vi "IQR Filter 3.vi"(9 "Z Values":dbl[](array[numeric]), 10 "Y Values":dbl[](array[numeric]), 11 "X Values":dbl[](array[numeric])) -> (1 "Z Vector":dbl[](array[numeric]), 2 "Y Vector":dbl[](array[numeric]), 3 "X Value":dbl[](array[numeric]))   [LabVIEW 2017]
uses:
  <vilib>/Analysis/NI_AALBase.lvlib
panel:
  out "Outliers":i32[](array[numeric])
  out "Higher Inner Fence":dbl
  out "Lower Inner Fence":dbl
  out "Interquartile Range":dbl
  out "Q1":dbl format="%.10f"
  out "median":dbl format="%.10f"
  out "Q3":dbl format="%.10f"
  out "X Histogram":T1(graph)
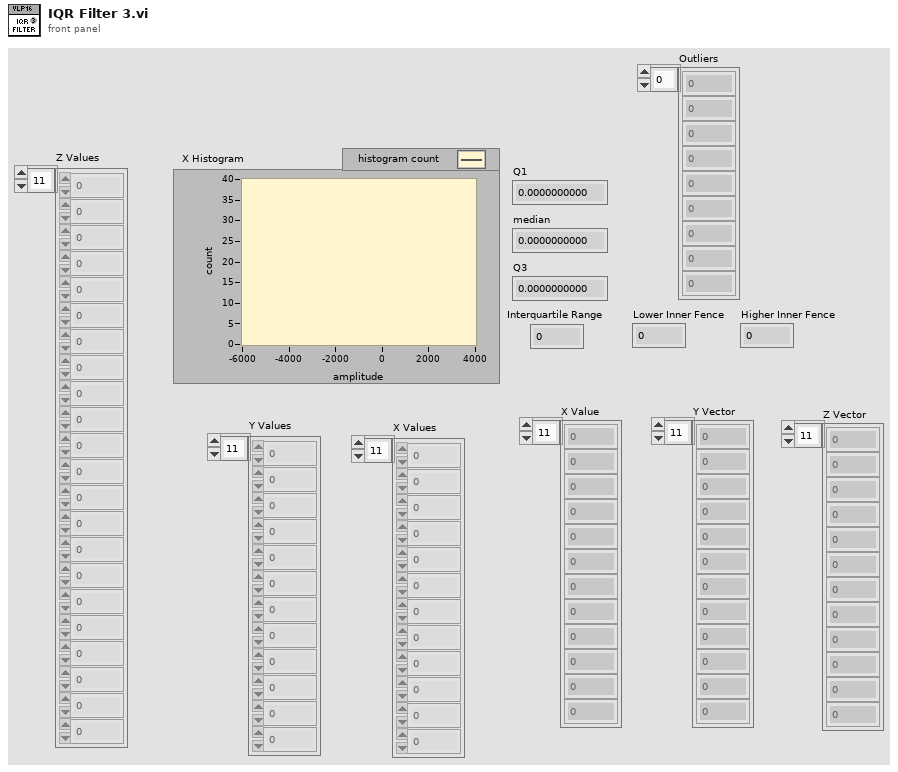
[diagram p1: front panel]
types:
  T1 = cluster{"X Values":dbl[], "Histogram: h(x)":i32[]}
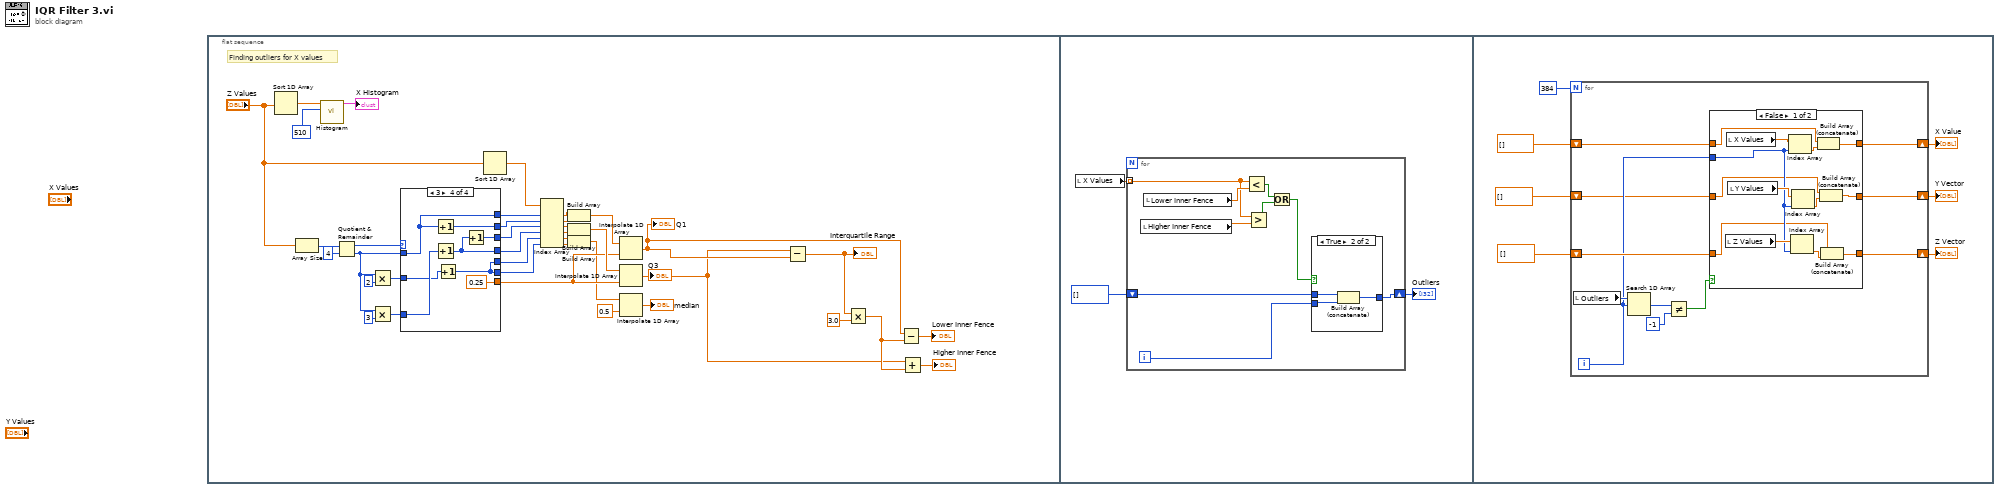
[diagram p0: block diagram]
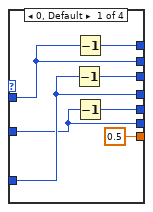
[diagram p2: hidden frame]
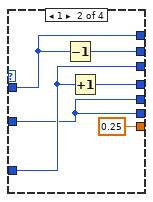
[diagram p3: hidden frame]
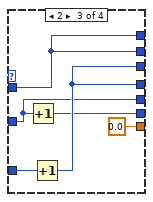
[diagram p4: hidden frame]
diagram:
  n1 = flat-sequence {
    frame #0 {
      # "Finding outliers for X values"
      n2 = Sort 1D Array(array="Z Values") -> (sorted array=w36:dbl[])
      n3 = Array Size(array="Z Values") -> (size(s)=w35:i32)
      n4 = call <vilib>:"Histogram.vi"("intervals"=510, "X"=w36) -> ("Histogram Graph"=→"X Histogram":T1)  [unwired: 6 in, 3 out]
      n5 = Quotient & Remainder(x=w35, y=4) -> (x-y*floor(x/y)=w33:i32, floor(x/y)=w14:i32)
      n6 = Multiply(x=w14, y=2) -> (x*y=w13:i32)
      n7 = Multiply(x=w14, y=3) -> (x*y=w20:i32)
      n8 = case shown="3" w33 {
        tunnel: w14 -> [w45 w50 w57 w64]
        tunnel: [w43 w50 w57 w64] -> w25
        tunnel: [w45 w47 w57 w65] -> w24
        tunnel: [w41 w49 w54 w62] -> w23
        tunnel: [w44 w48 w54 w60] -> w22
        tunnel: w20 -> [w44 w49 w56 w61]
        tunnel: [0.5 0.25 0.0 0.25] -> w19
        tunnel: w13 -> [w39 w46 w53 w59]
        tunnel: [w40 w46 w53 w58] -> w11
        tunnel: [w39 w46 w52 w58] -> w10
        frame 0, Default {
          n9 = Decrement(x=w44) -> (x-1=w41:i32)
          n10 = Decrement(x=w45) -> (x-1=w43:i32)
          n11 = Decrement(x=w39) -> (x-1=w40:i32)
        }
        frame 1 {
          n12 = Decrement(x=w50) -> (x-1=w47:i32)
          n13 = Increment(x=w49) -> (x+1=w48:i32)
        }
        frame 2 {
          n14 = Increment(x=w53) -> (x+1=w52:i32)
          n15 = Increment(x=w56) -> (x+1=w54:i32)
        }
        frame 3 {
          n16 = Increment(x=w64) -> (x+1=w65:i32)
          n17 = Increment(x=w61) -> (x+1=w60:i32)
          n18 = Increment(x=w59) -> (x+1=w58:i32)
          n19 = Increment(x=w60) -> (x+1=w62:i32)
        }
      }
      n20 = Sort 1D Array(array="Z Values") -> (sorted array=w32:dbl[])
      n21 = Index Array(array=w32, index #1=w25, index #2=w24, index #3=w23, index #4=w22, index #5=w11, index #6=w10) -> (element #1=w31:dbl, element #2=w30:dbl, element #3=w29:dbl, element #4=w28:dbl, element #5=w18:dbl, element #6=w17:dbl)
      n22 = Build Array(w31, w30) -> (w27:dbl[])
      n23 = Build Array(w29, w28) -> (w26:dbl[])
      n24 = Build Array(w18, w17) -> (w16:dbl[])
      n25 = Interpolate 1D Array(1:w19, 2:w27) -> (0:w4:dbl)
      "Q1" <- w4
      n26 = Interpolate 1D Array(1:w19, 2:w26) -> (0:w3:dbl)
      "Q3" <- w3
      n27 = Interpolate 1D Array(1:0.5 ("fractional index or x"), 2:w16) -> (0:→"median":dbl)
      n28 = Subtract(x=w3, y=w4) -> (x-y=w2:dbl)
      "Interquartile Range" <- w2
      n29 = Multiply(x=w2, y=3.0) -> (x*y=w7:dbl)
      n30 = Subtract(x=w4, y=w7) -> (x-y=→"Lower Inner Fence":dbl)
      n31 = Add(x=w3, y=w7) -> (x+y=→"Higher Inner Fence":dbl)
    }
    frame #1 {
      n32 = local read "X Values"() -> (w68:dbl[])
      n33 = for {
        tunnel: w68 -> [w73] mode=indexing
        shift-right: [w74] -> w66
        shift-left: i32[] [] -> [w76]
        i -> [w75]
        n34 = local read "Higher Inner Fence"() -> (w72:dbl)
        n35 = local read "Lower Inner Fence"() -> (w77:dbl)
        n36 = Less?(x=w73, y=w77) -> (x < y?=w71:bool)
        n37 = Greater?(x=w73, y=w72) -> (0:w70:bool)
        n38 = Or(x=w71, y=w70) -> (x .or. y?=w69:bool)
        n39 = case shown="True" w69 {
          tunnel: w76 -> [w78 w81]
          tunnel: w75 -> [_ w80]
          tunnel: [w78 w79] -> w74
          frame False {
          }
          frame True {
            n40 = Build Array (concatenate)(w81, w80) -> (w79:i32[])
          }
        }
      }
      "Outliers" <- w66
    }
    frame #2 {
      n41 = for {
        N: 384 -> [_]
        shift-right: [w94] -> w82
        shift-left: dbl[] [] -> [w95]
        shift-right: [w90] -> w83
        shift-left: dbl[] [] -> [w89]
        shift-right: [w92] -> w84
        shift-left: dbl[] [] -> [w93]
        i -> [w91]
        n42 = local read "Outliers"() -> (w99:i32[])
        n43 = Search 1D Array(1D array=w99, element=w91) -> (index of element=w98:i32)  [unwired: 1 in]
        n44 = Not Equal?(x=w98, y=-1) -> (x != y?=w96:bool)
        n45 = case shown="False" w96 {
          tunnel: w95 -> [w100 w115]
          tunnel: [w106 w115] -> w94
          tunnel: w93 -> [w102 w114]
          tunnel: [w112 w114] -> w92
          tunnel: w91 -> [w107 _]
          tunnel: [w108 w113] -> w90
          tunnel: w89 -> [w101 w113]
          frame False {
            n46 = local read "Z Values"() -> (w109:dbl[])
            n47 = local read "X Values"() -> (w111:dbl[])
            n48 = local read "Y Values"() -> (w110:dbl[])
            n49 = Index Array(array=w111, index=w107) -> (element=w103:dbl)
            n50 = Index Array(array=w109, index=w107) -> (element=w105:dbl)
            n51 = Index Array(array=w110, index=w107) -> (element=w104:dbl)
            n52 = Build Array (concatenate)(w102, w103) -> (w112:dbl[])
            n53 = Build Array (concatenate)(w101, w104) -> (w108:dbl[])
            n54 = Build Array (concatenate)(w100, w105) -> (w106:dbl[])
          }
          frame True {
          }
        }
      }
      "X Value" <- w84
      "Y Vector" <- w83
      "Z Vector" <- w82
    }
  }
